vi "Eval centre.vi"(0 "Xpos":refnum<vi>, 1 "Ypos":refnum<vi>, 2 "Zpos":refnum<vi>, 3 "Thetapos":refnum<vi>, 5 "VISA resource name":refnum<visa-resource-name>, 7 "X inc":dbl, 9 "Y inc":dbl, 11 "error in (no error)":errorcluster) -> (6 "VISA Refnum out":refnum<visa-resource-name>, 8 "Difference":dbl, 10 "Voltage":dbl[](graph), 13 "Mean":dbl, 14 "Std dev":dbl, 15 "error out":errorcluster)   [LabVIEW 2020]
uses:
  <vilib>/Analysis/NI_AALBase.lvlib
panel:
  out "Voltage 2":dbl(graph)
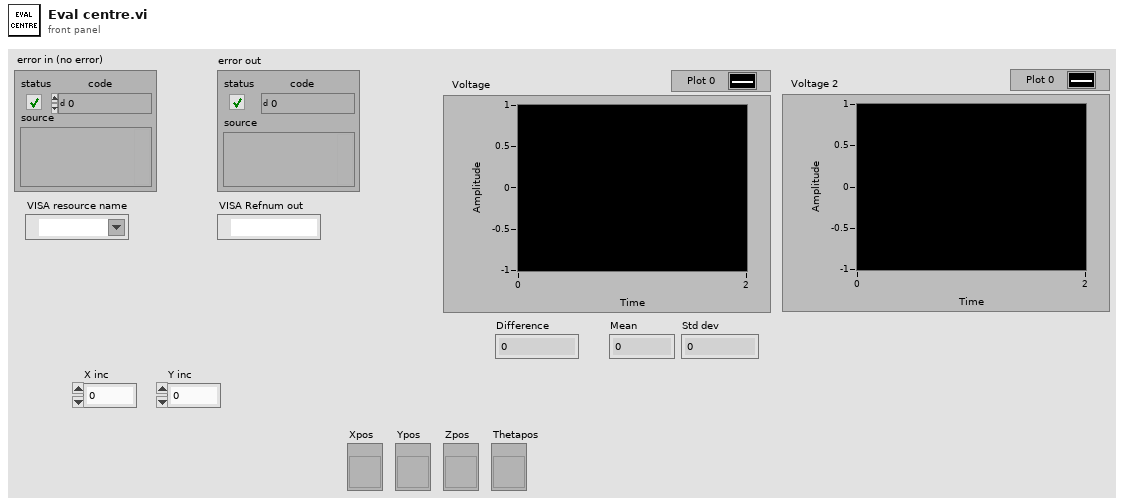
[diagram p1: front panel]
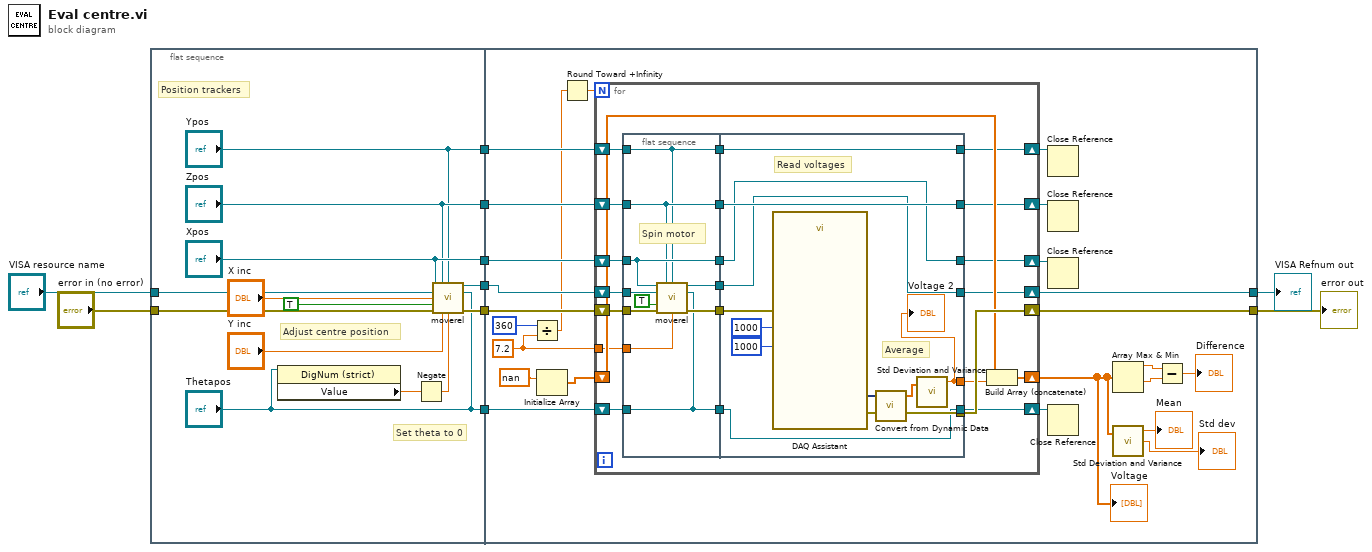
[diagram p0: block diagram]
diagram:
  n1 = flat-sequence {
    tunnel: [w19] -> w6
    tunnel: [w20] -> w5
    tunnel: ["Xpos"] -> w4
    tunnel: ["Zpos"] -> w3
    tunnel: ["Ypos"] -> w2
    tunnel: ["Thetapos"] -> w1
    tunnel: "error in (no error)" -> [w11]
    tunnel: "VISA resource name" -> [w12]
    tunnel: [w47] -> w7
    tunnel: [w46] -> w9
    tunnel: w1 -> [w34]
    tunnel: w2 -> [w35]
    tunnel: w3 -> [w36]
    tunnel: w4 -> [w37]
    tunnel: w5 -> [w44]
    tunnel: w6 -> [w45]
    frame #0 {
      # "Position trackers"
      # "Set theta to 0"
      # "Adjust centre position"
      n2 = property class="DigNum (strict)"(reference="Thetapos") -> ("Value"=w15:dbl)  [unwired: 1 in, 2 out]
      n3 = Negate(x=w15) -> (-x=w14:dbl)
      n4 = call "moverel.vi"("Xpos"="Xpos", "Zpos"="Zpos", "Ypos"="Ypos", "VISA resource name"=w12, "Thetapos"="Thetapos", "X increment"="X inc", "Theta on"=TRUE, "error in (no error)"=w11, "Y increment"="Y inc", "Theta inc"=w14) -> ("VISA Refnum out"=w20:refnum<visa-resource-name>, "error out"=w19:errorcluster)  [unwired: 4 in]
    }
    frame #1 {
      w29 = 7.2
      n5 = Divide(x=360, y=w29) -> (x/y=w27:dbl)
      n6 = Initialize Array(nan) -> (w25:dbl[])  [unwired: 1 in]
      n7 = Round Toward +Infinity(x=w27) -> (ceil(x): smallest int >= x=w26:dbl)
      n8 = for {
        N: w26 -> [_]
        shift-right: [w49] -> w47
        shift-left: w44 -> [w68]
        shift-right: [w67] -> w46
        shift-left: w45 -> [w69]
        shift-right: [w65] -> w38
        shift-left: w25 -> [w66]
        shift-right: [w50] -> w33
        shift-left: w35 -> [w59]
        shift-right: [w51] -> w32
        shift-left: w36 -> [w60]
        shift-right: [w52] -> w31
        shift-left: w37 -> [w61]
        shift-right: [w53] -> w30
        shift-left: w34 -> [w58]
        tunnel: w29 -> [w48]
        n9 = flat-sequence {
          tunnel: w69 -> [w78]
          tunnel: w68 -> [w79]
          tunnel: [w77] -> w63
          tunnel: [w76] -> w62
          tunnel: w61 -> [w73]
          tunnel: w60 -> [w72]
          tunnel: w59 -> [w71]
          tunnel: w58 -> [w74]
          tunnel: [w74] -> w57
          tunnel: [w73] -> w56
          tunnel: [w72] -> w55
          tunnel: [w71] -> w54
          tunnel: w48 -> [w70]
          tunnel: [w80] -> w64
          tunnel: [w87] -> w67
          tunnel: w63 -> [w86]
          tunnel: w62 -> [w82]
          tunnel: w57 -> [w81]
          tunnel: w56 -> [w83]
          tunnel: w55 -> [w84]
          tunnel: w54 -> [w85]
          tunnel: [w85] -> w50
          tunnel: [w84] -> w51
          tunnel: [w83] -> w52
          tunnel: [w81] -> w53
          tunnel: [w82] -> w49
          frame #0 {
            # "Spin motor"
            n10 = call "moverel.vi"("Xpos"=w73, "Zpos"=w72, "Ypos"=w71, "VISA resource name"=w79, "Thetapos"=w74, "Theta on"=TRUE, "error in (no error)"=w78, "Theta inc"=w70) -> ("VISA Refnum out"=w76:refnum<visa-resource-name>, "error out"=w77:errorcluster)  [unwired: 6 in]
          }
          frame #1 {
            # "Average"
            # "Read voltages"
            n11 = call "DAQ Assistant"("rate"=u16 1000, "number of samples"=u16 1000, "error in"=w86) -> ("data"=w90:dynamicdata, "error out"=w87:errorcluster)  [unwired: 14 in, 1 out]
            n12 = call "Convert from Dynamic Data"("Dynamic Data Type"=w90) -> ("Array"=w89:dbl[])  [unwired: 3 in]
            n13 = call <vilib>:"Std Deviation and Variance.vi"("X"=w89) -> ("mean"=w80:dbl)  [unwired: 1 in, 2 out]
            "Voltage 2" <- w80
          }
        }
        n14 = Build Array (concatenate)(w66, w64) -> (w65:dbl[])
      }
      "Voltage" <- w38
      n15 = Close Reference(reference=w33) -> ()  [unwired: 1 in, 1 out]
      n16 = Close Reference(reference=w32) -> ()  [unwired: 1 in, 1 out]
      n17 = Close Reference(reference=w31) -> ()  [unwired: 1 in, 1 out]
      n18 = Close Reference(reference=w30) -> ()  [unwired: 1 in, 1 out]
      n19 = Array Max & Min(array=w38) -> (max value=w43:dbl, min value=w41:dbl)  [unwired: 2 out]
      n20 = call <vilib>:"Std Deviation and Variance.vi"("X"=w38) -> ("mean"=→"Mean":dbl, "standard deviation"=→"Std dev":dbl)  [unwired: 1 in, 1 out]
      n21 = Subtract(x=w43, y=w41) -> (x-y=→"Difference":dbl)
    }
  }
  "error out" <- w9
  "VISA Refnum out" <- w7
